vi "Main.vi"() -> ()   [LabVIEW 2019]
doc: "The myRIO Project template acquires acceleration data from the onboard accelerometer and displays the changes of acceleration values in a waveform chart."
uses:
  <vilib>/myRIO/Instrument Drivers/Onboard IO/UART/typedef/VISA Configuration.ctl
  <vilib>/Instr/_visa.llb/VISA Configure Serial Port (Instr).vi
  <vilib>/myRIO/Instrument Drivers/Onboard IO/UART/UART.lvlib
panel:
  out "Distance":u16
  out "unsigned byte array":u8[](array[numeric])
  in  "Stop Button":bool
  out "x = y?":bool
  out "read buffer":string
  out "error out":errorcluster
  in  "error in (no error)":errorcluster
  out "Character Count":u32
  # "mm"
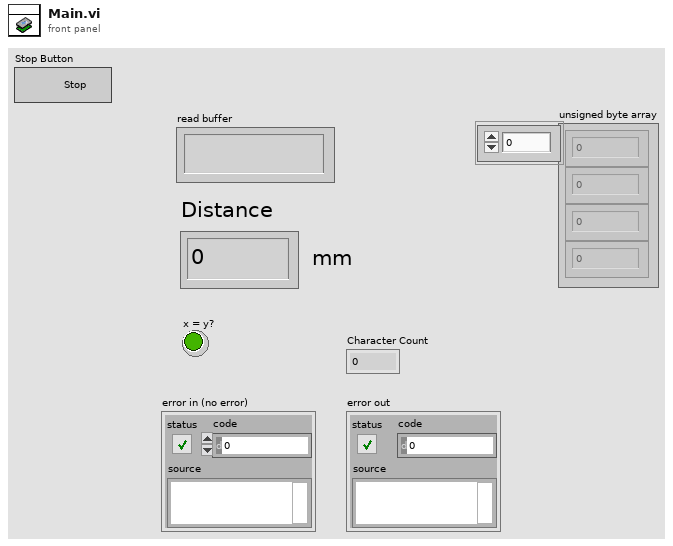
[diagram p1: front panel]
types:
  T1 = typedef "UART.lvlib/VISA Configuration.ctl" = cluster{"baud rate (9600)":u32, "data bits (8)":u16, "parity (0:none)":enum16{"None", "Odd", "Even", "Mark", "Space"}, "stop bits (10: 1 bit)":u16, "flow control (0:none)":u16, "termination char\n(0xA = '\\n' = LF) ":u8, "Enable Termination\nChar (T)":bool, "timeout (10sec)":u32}
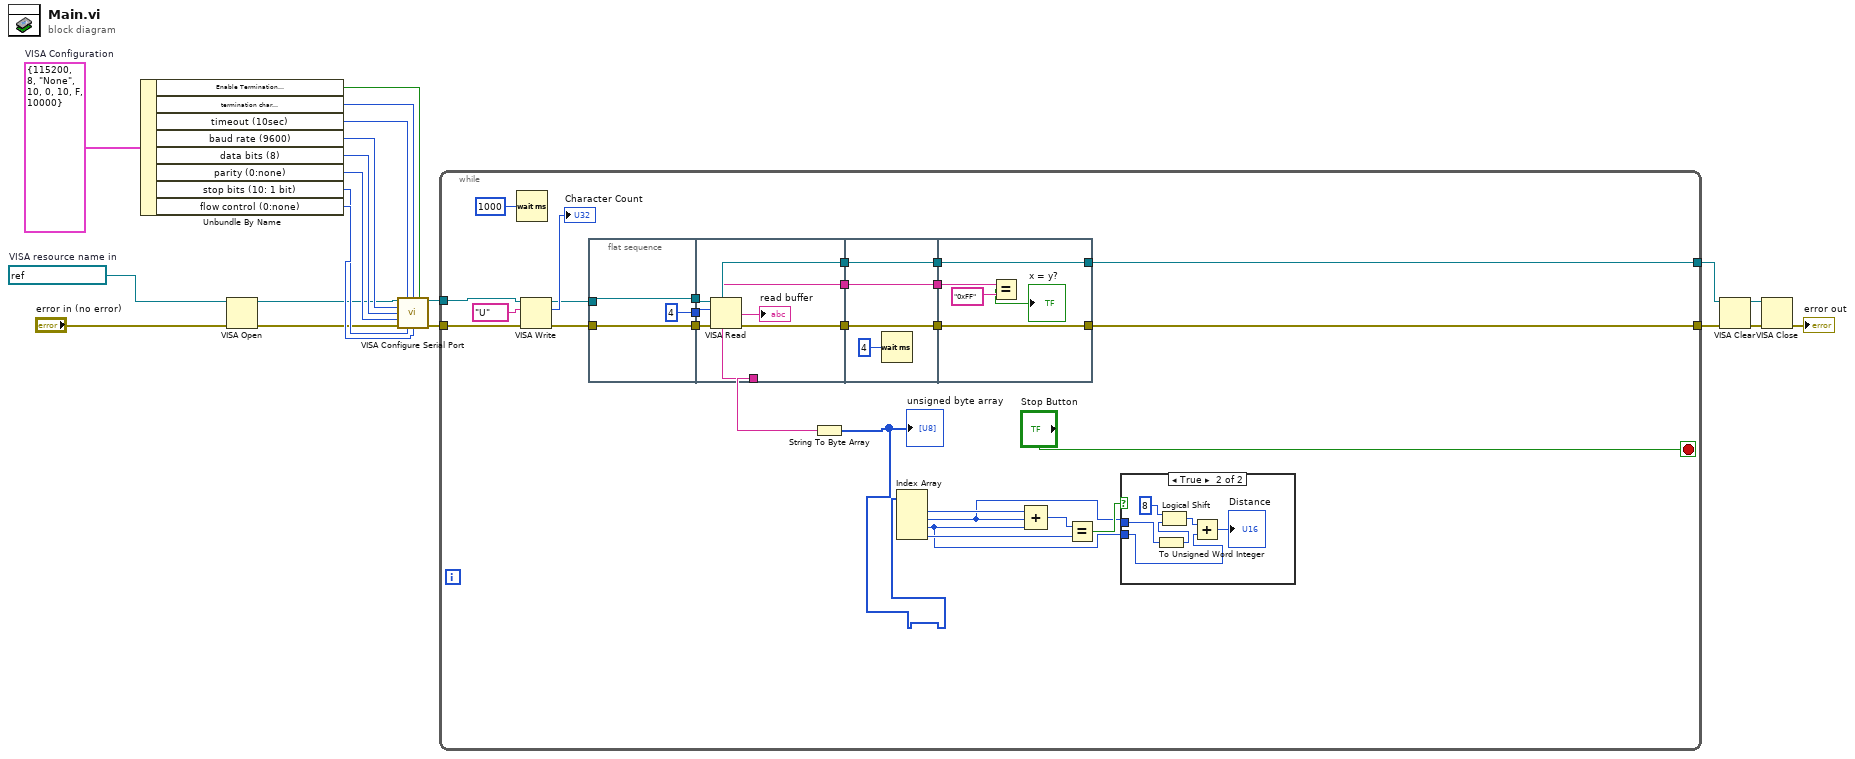
[diagram p0: block diagram]
diagram:
  w20 = T1 {"baud rate (9600)"=115200, "data bits (8)"=8, "parity (0:none)"=enum."None", "stop bits (10: 1 bit)"=10, "flow control (0:none)"=0, "termination char\n(0xA = '\\n' = LF) "=10, "Enable Termination\nChar (T)"=FALSE, "timeout (10sec)"=10000}  # VISA Configuration
  w6 = refnum<visa-resource-name> "ASRL1::INSTR"  # VISA resource name in
  n1 = Unbundle By Name(w20) -> ("Enable Termination\nChar (T)"=w17:bool, "termination char\n(0xA = '\\n' = LF)"=w16:u8, "timeout (10sec)"=w15:u32, "baud rate (9600)"=w10:u32, "data bits (8)"=w11:u16, "parity (0:none)"=w12:enum16{"None", "Odd", "Even", "Mark", "Space"}, "stop bits (10: 1 bit)"=w13:u16, "flow control (0:none)"=w14:u16)
  n2 = VISA Open(error in (no error)="error in (no error)", VISA resource name=w6) -> (VISA resource name=w3:refnum<visa-resource-name>, error out=w4:errorcluster)  [unwired: 3 in]
  n3 = call-poly "VISA Configure Serial Port"("VISA resource name"=w3, "timeout (10sec)"=w15, "termination char\n(0xA = '\\n' = LF)"=w16, "Enable Termination\nChar (T)"=w17, "baud rate (9600)"=w10, "data bits (8)"=w11, "parity (0:none)"=w12, "error in (no error)"=w4, "stop bits (10: 1 bit)"=w13, "flow control (0:none)"=w14) -> ("VISA resource name out"=w19:refnum<visa-resource-name>, "error out"=w18:errorcluster)  [unwired: 4 in]
  n4 = while {
    tunnel: w18 -> [w35]
    tunnel: [w31] -> w1
    tunnel: w19 -> [w36]
    tunnel: [w32] -> w2
    stop <- "Stop Button" stop-if-true
    n5 = Wait (ms)(milliseconds to wait=u32 1000) -> ()  [unwired: 1 out]
    n6 = VISA Write(VISA resource name=w36, write buffer="U" ("Characters to Write"), error in (no error)=w35) -> (VISA resource name out=w34:refnum<visa-resource-name>, return count=→"Character Count":u32, error out=w33:errorcluster)
    n7 = flat-sequence {
      tunnel: w33 -> [w55]
      tunnel: w34 -> [w56]
      tunnel: [w56] -> w47
      tunnel: [w55] -> w46
      tunnel: [u32 4 ("byte count")] -> w45
      tunnel: w47 -> [w62]
      tunnel: w46 -> [w61]
      tunnel: [w60] -> w44
      tunnel: [w59] -> w43
      tunnel: [w57] -> w42
      tunnel: w45 -> [w58]
      tunnel: [w57] -> w28
      tunnel: w44 -> [w66]
      tunnel: w43 -> [w65]
      tunnel: [w66] -> w41
      tunnel: [w65] -> w40
      tunnel: w42 -> [w63]
      tunnel: [w63] -> w39
      tunnel: [w70] -> w31
      tunnel: [w71] -> w32
      tunnel: w41 -> [w71]
      tunnel: w40 -> [w70]
      tunnel: w39 -> [w69]
      frame #0 {
      }
      frame #1 {
        n8 = VISA Read(VISA resource name=w62, byte count=w58, error in (no error)=w61) -> (VISA resource name out=w60:refnum<visa-resource-name>, read buffer=w57:string, error out=w59:errorcluster)  [unwired: 1 out]
        "read buffer" <- w57
      }
      frame #2 {
        n9 = Wait (ms)(milliseconds to wait=u32 4) -> ()  [unwired: 1 out]
      }
      frame #3 {
        n10 = Equal?(x=w69, y="0xFF") -> (x = y?=→"x = y?":bool)
      }
    }
    n11 = String To Byte Array(string=w28) -> (unsigned byte array=w21:u8[])
    "unsigned byte array" <- w21
    n12 = Index Array(array=w21) -> (element #1=w27:u8, element #2=w23:u8, element #3=w22:u8, element #4=w25:u8)  [unwired: 4 in]
    n13 = Compound Arithmetic op=ADD(w27, w23, w22) -> (w26:u8)
    n14 = Equal?(x=w26, y=w25) -> (x = y?=w24:bool)
    n15 = case shown="True" w24 {
      tunnel: w23 -> [_ w49]
      tunnel: w22 -> [_ w51]
      frame False {
      }
      frame True {
        n16 = To Unsigned Word Integer(number=w49) -> (unsigned 16bit integer=w48:u16)
        n17 = Logical Shift(y=u8 8 ("x"), x=w48) -> (x << y=w52:u16)
        n18 = Add(x=w52, y=w51) -> (x+y=→"Distance":u16)
      }
    }
  }
  n19 = VISA Clear(VISA resource name=w2, error in (no error)=w1) -> (VISA resource name out=w9:refnum<visa-resource-name>, error out=w8:errorcluster)
  n20 = VISA Close(VISA resource name=w9, error in (no error)=w8) -> (error out=→"error out":errorcluster)
